vi "Thevenin to PT.vi"(0 "path in":path=path "C:/Data/XYZ DATA/XYZ999/FPL_R1/54.0mm.calib", 11 "error in (no error)":errorcluster) -> (15 "error out":errorcluster)   [LabVIEW 2015]
uses:
  Utility VIs/Math VIs/Z to dB, degrees (1D).vi
panel:
  in  "appended path":path=path "C:/Data/XYZ DATA/XYZ999/FPL_R1"
  out "XY Graph":T1(graph)
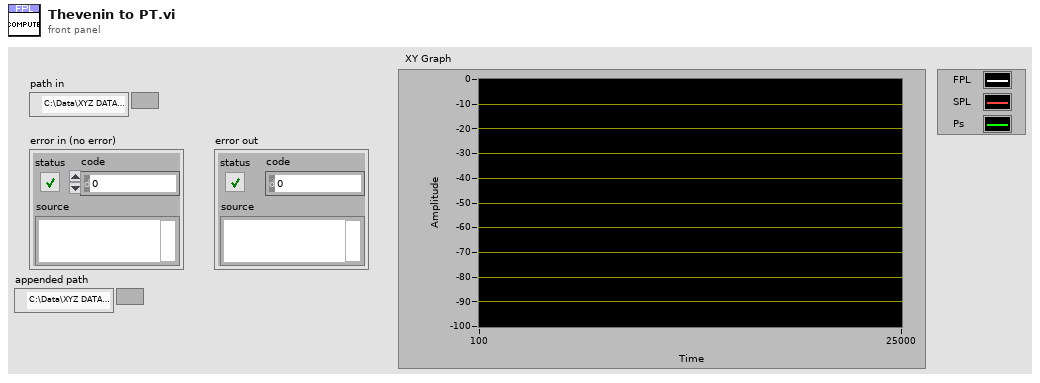
[diagram p1: front panel]
types:
  T1 = cluster{"Frequency (Hz)":dbl[], "Magnitude (dB)":dbl[]}[]
  T2 = cluster{"Frequency (Hz)":dbl[], "Magnitude (dB)":dbl[]}
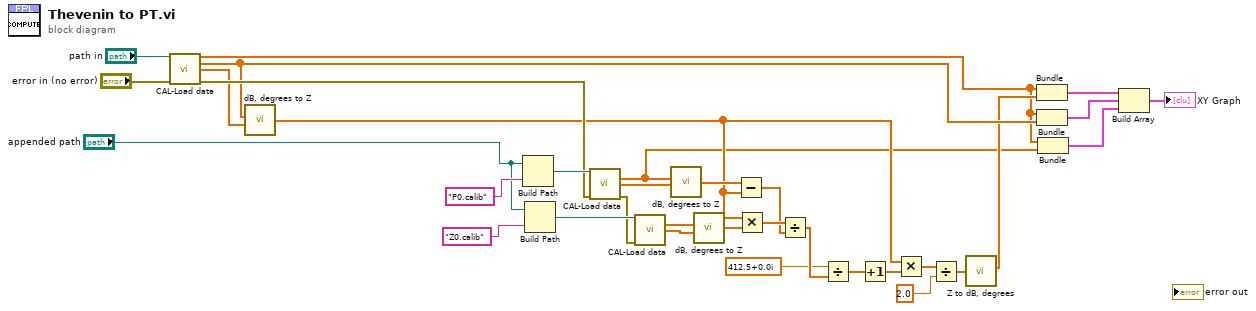
[diagram p0: block diagram]
diagram:
  n1 = call "CAL-Load data.vi"("user path"="path in", "error in (no error)"="error in (no error)") -> ("Frequency (Hz)"=w5:dbl[], "Mag"=w8:dbl[], "Phase"=w23:dbl[], "error out"=w28:errorcluster)  [unwired: 6 in, 4 out]
  n2 = call "dB, degrees to Z.vi"("Magnitude (dB)"=w8, "Phase (degrees)"=w23) -> ("Z"=w11:cdb[])  [unwired: 5 in]
  n3 = Build Path(base path="appended path", name or relative path="P0.calib") -> (appended path=w30:path)
  n4 = Build Path(base path="appended path", name or relative path="Z0.calib") -> (appended path=w29:path)
  n5 = call "CAL-Load data.vi"("user path"=w30, "error in (no error)"=w28) -> ("Mag"=w4:dbl[], "Phase"=w26:dbl[], "error out"=w27:errorcluster)  [unwired: 6 in, 5 out]
  n6 = call "CAL-Load data.vi"("user path"=w29, "error in (no error)"=w27) -> ("Mag"=w25:dbl[], "Phase"=w24:dbl[])  [unwired: 6 in, 6 out]
  n7 = call "dB, degrees to Z.vi"("Magnitude (dB)"=w4, "Phase (degrees)"=w26) -> ("Z"=w22:cdb[])  [unwired: 5 in]
  n8 = call "dB, degrees to Z.vi"("Magnitude (dB)"=w25, "Phase (degrees)"=w24) -> ("Z"=w18:cdb[])  [unwired: 5 in]
  n9 = Subtract(x=w22, y=w11) -> (x-y=w20:cdb[])
  n10 = Multiply(x=w11, y=w18) -> (x*y=w21:cdb[])
  n11 = Divide(x=w21, y=w20) -> (x/y=w19:cdb[])
  n12 = Divide(x=cdb 412.5+0.0i, y=w19) -> (x/y=w17:cdb[])
  n13 = Increment(x=w17) -> (x+1=w16:cdb[])
  n14 = Multiply(x=w11, y=w16) -> (x*y=w15:cdb[])
  n15 = Divide(x=w15, y=2.0) -> (x/y=w13:cdb[])
  n16 = call-poly "Z to dB, degrees.vi"("Z"=w13) -> ("Magnitude (dB)"=w7:dbl[])  [unwired: 5 in, 1 out]
  n17 = Bundle("Frequency (Hz)"=w5, "Magnitude (dB)"=w7) -> (w12:T2)  [unwired: 1 in]
  n18 = Bundle("Frequency (Hz)"=w5, "Mag"=w8) -> (w9:cluster{"Frequency (Hz)":dbl[], "Mag":dbl[]})  [unwired: 1 in]
  n19 = Bundle("Frequency (Hz)"=w5, "Mag"=w4) -> (w3:cluster{"Frequency (Hz)":dbl[], "Mag":dbl[]})  [unwired: 1 in]
  n20 = Build Array(w12, w9, w3) -> (→"XY Graph":cluster{"Frequency (Hz)":dbl[], "Mag":dbl[]}[])
